vi "Drive Chassies process.vi"(0 "error in":errorcluster) -> ()   [LabVIEW 2012]
uses:
  Drive Global Data.vi
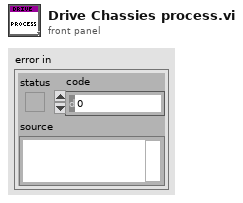
[diagram p1: front panel]
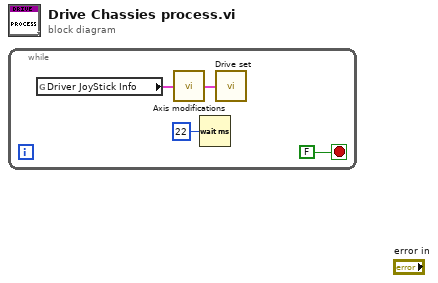
[diagram p0: block diagram]
diagram:
  n1 = while {
    stop <- FALSE stop-if-true
    n2 = global read "Drive Global Data.vi" "Driver JoyStick Info"() -> (w4:cluster{"Slow Drive?":bool, "Axisses":dbl[]})
    n3 = call "Axis modifications.vi"("Driver JoyStick Info"=w4) -> ("Driver JoyStick Info Out"=w3:cluster{"Slow Drive?":bool, "Axisses":dbl[]})
    n4 = Wait (ms)(milliseconds to wait=u32 22) -> ()  [unwired: 1 out]
    n5 = call "Drive set.vi"("Driver JoyStick Info"=w3) -> ()
  }
